vi "Make Component String.vi"(11 "Constructor String Parser":T1) -> (2 "Failed Assert?":bool, 3 "Component String":string)   [LabVIEW 2020, in "Stream.lvlib" / "URLPattern.lvclass"]
uses:
  URLPattern.lvclass
  Token Type.ctl
  Token.ctl
  URL Pattern Init.ctl
  Parser State.ctl
  Constructor String Parser.ctl
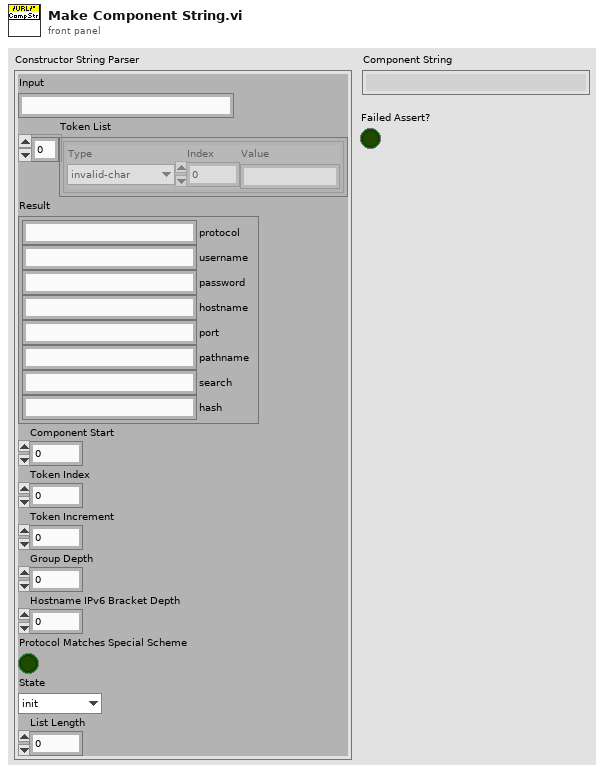
[diagram p1: front panel]
types:
  T1 = typedef "Stream.lvlib/URLPattern.lvclass/Constructor String Parser.ctl" = cluster{"Input":string, "Token List":T2[], "Result":T4, "Component Start":i32, "Token Index":i32, "Token Increment":i32, "Group Depth":i32, "Hostname IPv6 Bracket Depth":i32, "Protocol Matches Special Scheme":bool, "State":T5, "List Length":i32}
  T2 = typedef "Stream.lvlib/URLPattern.lvclass/Token.ctl" = cluster{"Type":T3, "Index":i32, "Value":string}
  T3 = typedef "Stream.lvlib/URLPattern.lvclass/Token Type.ctl" = enum16{"invalid-char", "open", "close", "regexp", "name", "char", "escaped-char", "other-modifier", "asterisk", "end"}
  T4 = typedef "Stream.lvlib/URLPattern.lvclass/URL Pattern Init.ctl" = cluster{"protocol":string, "username":string, "password":string, "hostname":string, "port":string, "pathname":string, "search":string, "hash":string}
  T5 = typedef "Stream.lvlib/URLPattern.lvclass/Parser State.ctl" = enum16{"init", "protocol", "authority", "username", "password", "hostname", "port", "pathname", "search", "hash", "done"}
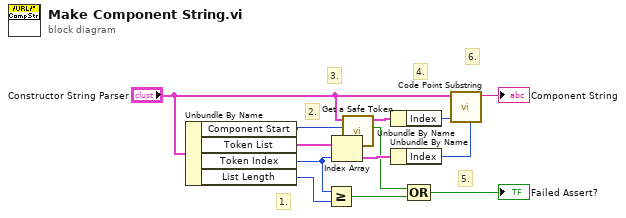
[diagram p0: block diagram]
diagram:
  # "6."
  # "5."
  # "4."
  # "3."
  # "2."
  # "1."
  n1 = Unbundle By Name("Constructor String Parser") -> ("Component Start"=w10:i32, "Token List"=w12:T2[], "Token Index"=w11:i32, "List Length"=w13:i32)
  n2 = Greater Or Equal?(x=w11, y=w13) -> (x >= y?=w7:bool)
  n3 = Index Array(array=w12, index=w11) -> (element=w8:T2)
  n4 = call "Get a Safe Token.vi"("Index"=w10, "Constructor String Parser"="Constructor String Parser") -> ("Failed Assert?"=w6:bool, "Token"=w9:T2)  [unwired: 8 in]
  n5 = Unbundle By Name(w9) -> ("Index"=w3:i32)
  n6 = Unbundle By Name(w8) -> ("Index"=w2:i32)
  n7 = Compound Arithmetic op=OR(w6, w7) -> (→"Failed Assert?":bool)
  n8 = call "Code Point Substring.vi"("End"=w2, "Start"=w3, "Constructor String Parser"="Constructor String Parser") -> ("Substring"=→"Component String":string)  [unwired: 8 in]
